vi "clFile_readFromString.vi"(11 "String":string) -> (2 "clFileReader.lvclass":refnum<class "clFileReader.lvclass">, 3 "clFile.lvclass":refnum<class "clFile.lvclass">)   [LabVIEW 2021, in "vi_lib.lvlib" / "clFile.lvclass"]
uses:
  clFile.lvclass
  clFile.lvclass/clFile.ctl
  clFileReader/clFileReader.lvclass
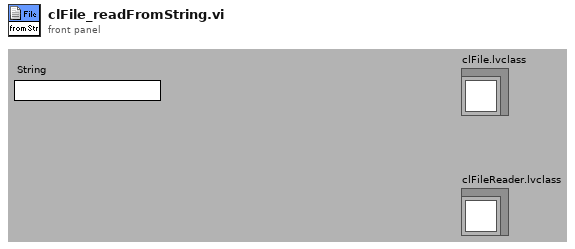
[diagram p1: front panel]
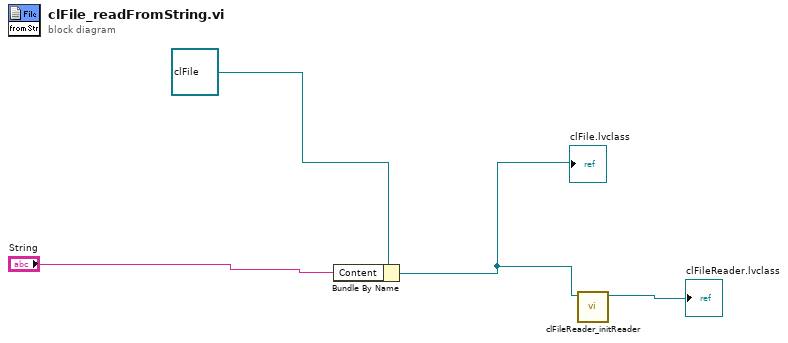
[diagram p0: block diagram]
diagram:
  n1 = Bundle By Name(cluster=refnum<class "clFile.lvclass"> refnum ("clFile.lvclass"), "Content"="String") -> (w2:refnum<class "clFile.lvclass">)
  "clFile.lvclass" <- w2
  n2 = call "clFileReader_initReader.vi"("clFile.lvclass"=w2) -> ("clFileReader.lvclass"=→"clFileReader.lvclass":refnum<class "clFileReader.lvclass">)  [unwired: 2 in, 8 out]
